vi "UpdateCurveData.vi"(3 "Mouse Position":cluster{"X":i32, "Y":i32}, 4 "Curve Data":cluster{i16, i16}[](array[cluster])) -> (0 "Refresh Curve Data":cluster{i16, i16}[](array[cluster]), 1 "Curve Data Out":cluster{i16, i16}[](array[cluster]))   [LabVIEW 2016]
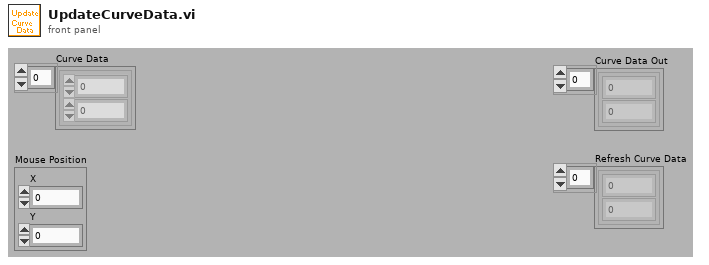
[diagram p1: front panel]
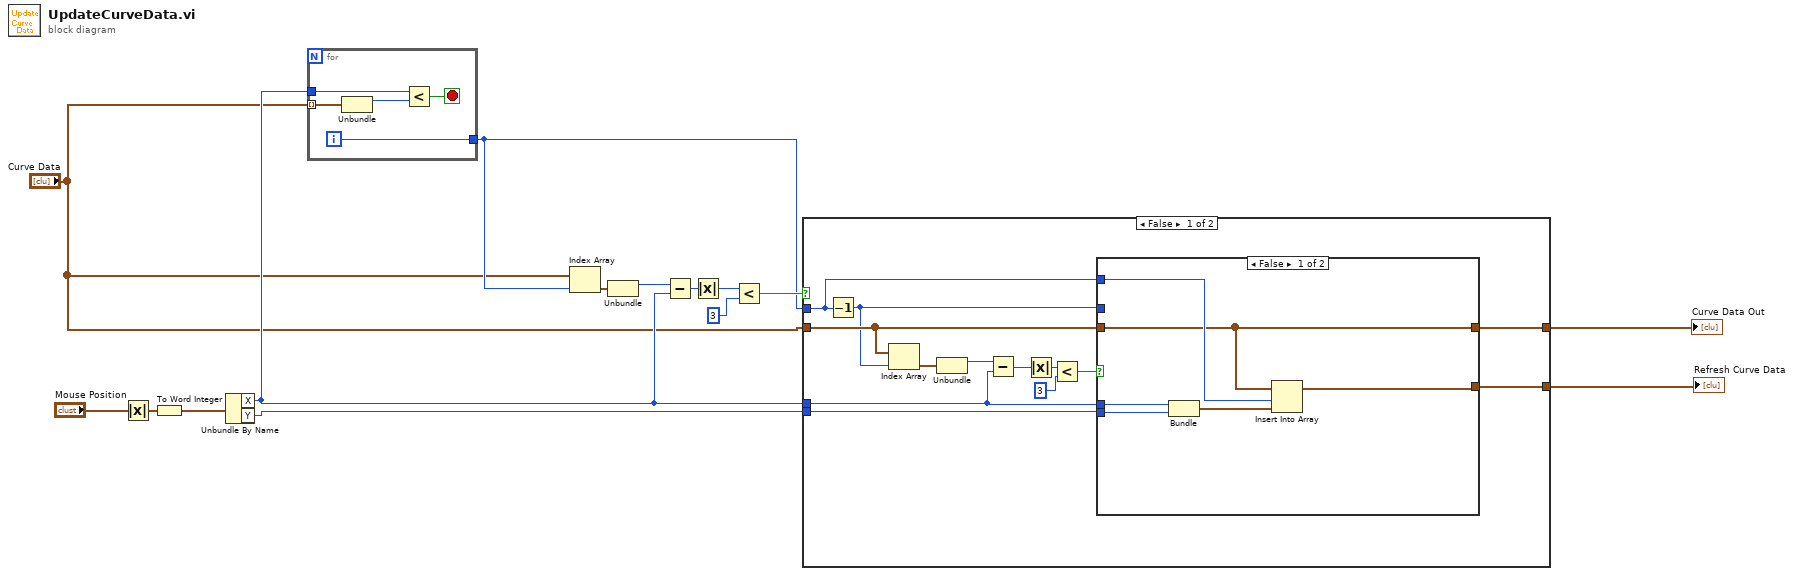
[diagram p0: block diagram]
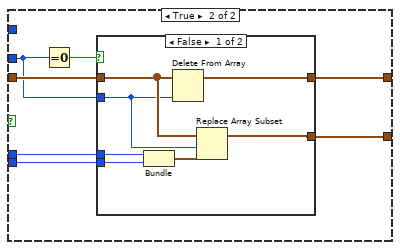
[diagram p2: hidden frame]
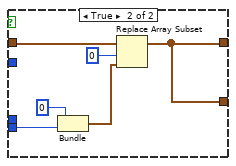
[diagram p3: hidden frame]
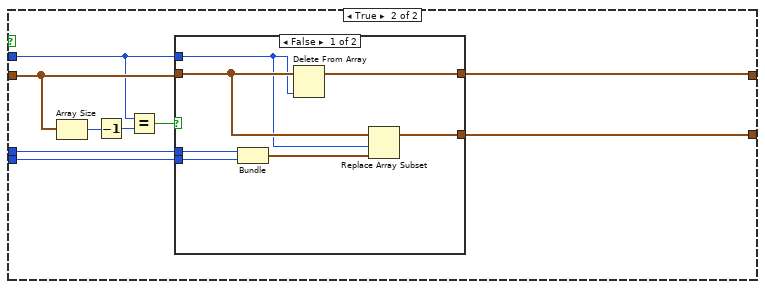
[diagram p4: hidden frame]
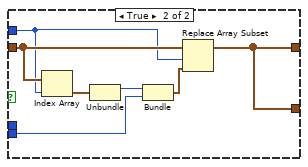
[diagram p5: hidden frame]
diagram:
  n1 = Absolute Value(x="Mouse Position") -> (abs(x)=w8:cluster{"X":i32, "Y":i32})
  n2 = To Word Integer(number=w8) -> (16bit integer=w4:cluster{"X":i16, "Y":i16})
  n3 = Unbundle By Name(w4) -> ("X"=w6:i16, "Y"=w7:i16)
  n4 = for {
    tunnel: "Curve Data" -> [w20] mode=indexing
    tunnel: w6 -> [w19]
    tunnel: [w17] -> w5
    i -> [w17]
    stop <- w16 stop-if-true
    n5 = Unbundle(w20) -> (w18:i16)  [unwired: 1 out]
    n6 = Less?(x=w19, y=w18) -> (x < y?=w16:bool)
  }
  n7 = Index Array(array="Curve Data", index=w5) -> (element=w9:cluster{i16, i16})
  n8 = Unbundle(w9) -> (w12:i16)  [unwired: 1 out]
  n9 = Subtract(x=w12, y=w6) -> (x-y=w13:i16)
  n10 = Absolute Value(x=w13) -> (abs(x)=w14:i16)
  n11 = Less?(x=w14, y=3) -> (x < y?=w10:bool)
  n12 = case shown="False" w10 {
    tunnel: "Curve Data" -> [w29 w66]
    tunnel: [w28 w67] -> w3
    tunnel: w5 -> [w23 w62]
    tunnel: w7 -> [w26 w64]
    tunnel: w6 -> [w22 w61]
    tunnel: [w21 w60] -> w1
    frame False {
      n13 = Decrement(x=w23) -> (x-1=w27:i32)
      n14 = Index Array(array=w29, index=w27) -> (element=w32:cluster{i16, i16})
      n15 = Unbundle(w32) -> (w24:i16)  [unwired: 1 out]
      n16 = Subtract(x=w24, y=w22) -> (x-y=w31:i16)
      n17 = Absolute Value(x=w31) -> (abs(x)=w30:i16)
      n18 = Less?(x=w30, y=3) -> (x < y?=w25:bool)
      n19 = case shown="False" w25 {
        tunnel: w29 -> [w35 w45]
        tunnel: [w35 w44] -> w28
        tunnel: w27 -> [_ w42]
        tunnel: w26 -> [w37 w43]
        tunnel: w23 -> [w39 _]
        tunnel: w22 -> [w38 w41]
        tunnel: [w34 w40] -> w21
        frame False {
          n20 = Bundle("X"=w38, "Y"=w37) -> (w36:cluster{"X":i16, "Y":i16})  [unwired: 1 out]
          n21 = Insert Into Array(array=w35, index=w39, new element=w36) -> (w34:cluster{i16, i16}[])
        }
        frame True {
          n22 = Equal To 0?(x=w42) -> (x = 0?=w46:bool)
          n23 = case shown="False" w46 {
            tunnel: w42 -> [w49 _]
            tunnel: w45 -> [w50 w57]
            tunnel: [w53 w54] -> w44
            tunnel: w43 -> [w51 w59]
            tunnel: w41 -> [w52 _]
            tunnel: [w47 w54] -> w40
            frame False {
              n24 = Bundle("X"=w52, "Y"=w51) -> (w48:cluster{"X":i16, "Y":i16})  [unwired: 1 out]
              n25 = Delete From Array(array=w50, index=w49) -> (array with subset deleted=w53:cluster{i16, i16}[])  [unwired: 1 in, 1 out]
              n26 = Replace Array Subset(array=w50, new element=w48, index=w49) -> (w47:cluster{i16, i16}[])
            }
            frame True {
              n27 = Bundle("y"=i16 0, "Y"=w59) -> (w58:cluster{"y":i16, "Y":i16})  [unwired: 1 out]
              n28 = Replace Array Subset(array=w57, new element=w58, index=0 ("索引")) -> (w54:cluster{i16, i16}[])
            }
          }
        }
      }
    }
    frame True {
      n29 = Array Size(array=w66) -> (size(s)=w65:i32)
      n30 = Decrement(x=w65) -> (x-1=w63:i32)
      n31 = Equal?(x=w62, y=w63) -> (x = y?=w68:bool)
      n32 = case shown="False" w68 {
        tunnel: w66 -> [w74 w81]
        tunnel: [w75 w76] -> w67
        tunnel: w62 -> [w73 w80]
        tunnel: w64 -> [w70 w77]
        tunnel: w61 -> [w71 _]
        tunnel: [w72 w76] -> w60
        frame False {
          n33 = Bundle("X"=w71, "Y"=w70) -> (w69:cluster{"X":i16, "Y":i16})  [unwired: 1 out]
          n34 = Delete From Array(array=w74, index=w73) -> (array with subset deleted=w75:cluster{i16, i16}[])  [unwired: 1 in, 1 out]
          n35 = Replace Array Subset(array=w74, new element=w69, index=w73) -> (w72:cluster{i16, i16}[])
        }
        frame True {
          n36 = Index Array(array=w81, index=w80) -> (element=w79:cluster{i16, i16})
          n37 = Unbundle(w79) -> (w78:i16)  [unwired: 1 out]
          n38 = Bundle(w78, "Y"=w77) -> (w82:cluster{i16, "Y":i16})  [unwired: 1 out]
          n39 = Replace Array Subset(array=w81, new element=w82, index=w80) -> (w76:cluster{i16, i16}[])
        }
      }
    }
  }
  "Curve Data Out" <- w3
  "Refresh Curve Data" <- w1
